vi "Set Up Data Repo.vi"(8 "error in (no error)":errorcluster, 11 "Application in":refnum<class "Application.lvclass">) -> (0 "error out":errorcluster, 3 "Application out":refnum<class "Application.lvclass">)   [LabVIEW 2017, in "Application.lvlib" / "Application.lvclass"]
doc: "Set up the required data header information in the repo."
uses:
  Application.lvclass
  <vilib>/TSS/ACRObat Test Framework/Core Launcher/Core Manager Methods -- Enum.ctl
  <vilib>/TSS/ACRObat Test Framework/Core Launcher/Core Launcher.lvlib
  <vilib>/TSS/ACRObat Test Framework/Classes/Data/Data Repo/Class/Data Repo.lvclass
  Test Recipe/Class/Test Recipe.lvclass
  Station Config/Class/Station Config.lvclass
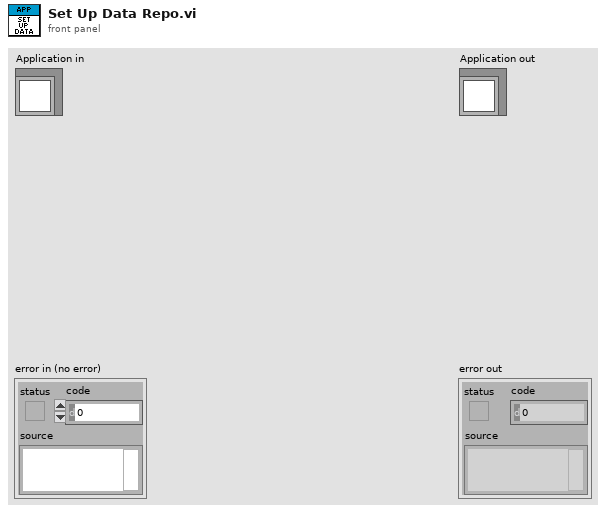
[diagram p1: front panel]
types:
  T1 = typedef "Core Launcher.lvlib/Core Manager Methods -- Enum.ctl" = enum16{"Spawn Objects", "Get Objects", "Destroy Objects"}
  T2 = cluster{"Serial":string, "DateCode":string, "MachID":string, "OperatorID":string, "PartNumber":string, "RecipeFileRev":string, "SoftwareRev":string, "LogField1":string, "LogField2":string, "LogField3":string, "OpMode":string, "PartFailCode":string, "MachineFailCode":string, "Position":string}
  T3 = typedef "Application.lvlib/App Properties.lvclass/Class Properties -- Cluster.ctl" = cluster{"UUT Info":T4[], "Test Information":refnum<vi>, "Gold Board":refnum<class "Golden Board.lvclass">, "Test Recipe":refnum<class "Test Recipe.lvclass">, "Instruments":refnum<class "Instrument.lvclass">[], "Mode":T5, "Test Results":T6[], "Station Config":refnum<class "Station Config.lvclass">, "Variable Engine":refnum<class "Variable Engine.lvclass">}
  T4 = typedef "Application.lvlib/App Properties.lvclass/UUT Reference -- Cluster.ctl" = cluster{"Serial Number Reference":refnum<vi>, "Status Message Reference":refnum<vi>}
  T5 = typedef "Application.lvlib/Application.lvclass/Op Mode -- Enum.ctl" = u16
  T6 = typedef "Application.lvlib/App Properties.lvclass/Test Result -- Cluster.ctl" = cluster{"Position":i32, "Pass":bool, "Fail Codes":string}
  T7 = typedef "Station Config.lvlib/Station Config.lvclass/Station Settings -- Cluster.ctl" = cluster{"Description":string, "ID":string}
  T8 = typedef "Application.lvlib/Application.lvclass/Test Info -- Cluster.ctl" = cluster{"Time / Date":string, "Operator ID":string, "Material":string, "Log Field":string, "Test Time":string, "Software Revision":string}
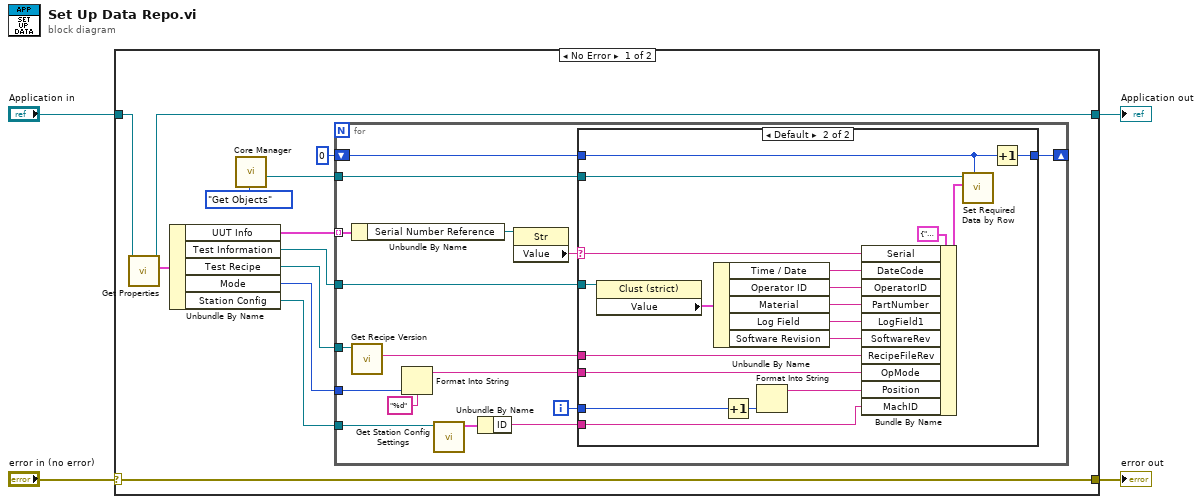
[diagram p0: block diagram]
diagram:
  n1 = case shown="No Error" "error in (no error)" {
    selector: "error in (no error)" -> [w16 w54]
    tunnel: [w16 w54] -> w3
    tunnel: [w14 w53] -> w1
    tunnel: "Application in" -> [w15 w53]
    frame No Error {
      n2 = call "Get Properties.vi"("Acrobat Template in"=w15) -> ("Class Properties"=w13:T3, "Acrobat Template out"=w14:refnum<class "Application.lvclass">)  [unwired: 8 in, 1 out]
      n3 = Unbundle By Name(w13) -> ("UUT Info"=w11:T4[], "Test Information"=w10:refnum<vi>, "Test Recipe"=w7:refnum<class "Test Recipe.lvclass">, "Mode"=w6:T5, "Station Config"=w5:refnum<class "Station Config.lvclass">)
      n4 = call <vilib>:"Core Manager.vi"("Method"=Core_Manager_Methods_--_Enum."Get Objects") -> ("Data Repo"=w12:refnum<class "Data Repo.lvclass">)  [unwired: 6 in, 4 out]
      n5 = for {
        tunnel: w12 -> [w32]
        tunnel: w11 -> [w29] mode=indexing
        tunnel: w10 -> [w30]
        shift-right: [w25] -> _
        shift-left: 0 -> [w26]
        tunnel: w7 -> [w24]
        tunnel: w6 -> [w22]
        tunnel: w5 -> [w19]
        i -> [w27]
        n6 = Unbundle By Name(w29) -> ("Serial Number Reference"=w28:refnum<vi>)
        n7 = call "Get Recipe Version.vi"("Test Recipe in"=w24) -> ("Test Recipe Version"=w23:string)  [unwired: 8 in, 2 out]
        n8 = Format Into String(format string="%d", w22) -> (resulting string=w20:string)  [unwired: 2 in, 1 out]
        n9 = call "Get Station Config Settings.vi"("Station Config in"=w19) -> ("Station Settings"=w18:T7)  [unwired: 9 in, 1 out]
        n10 = Unbundle By Name(w18) -> ("ID"=w17:string)
        n11 = property class="Str"(reference=w28) -> ("Value"=w31:string)  [unwired: 1 in, 2 out]
        n12 = case shown="Default" w31 {
          selector: w31 -> [_ w50]
          tunnel: w32 -> [_ w52]
          tunnel: w30 -> [_ w49]
          tunnel: w27 -> [_ w42]
          tunnel: w26 -> [w33 w39]
          tunnel: [w33 w38] -> w25
          tunnel: w23 -> [_ w36]
          tunnel: w20 -> [_ w37]
          tunnel: w17 -> [_ w34]
          frame "" {
          }
          frame Default {
            n13 = property class="Clust (strict)"(reference=w49) -> ("Value"=w47:T8)  [unwired: 1 in, 2 out]
            n14 = Unbundle By Name(w47) -> ("Time / Date"=w46:string, "Operator ID"=w45:string, "Material"=w44:string, "Log Field"=w43:string, "Software Revision"=w35:string)
            n15 = Increment(x=w42) -> (x+1=w40:i32)
            n16 = Format Into String(w40) -> (resulting string=w41:string)  [unwired: 3 in, 1 out]
            n17 = Bundle By Name(cluster=T2 {"Serial"="", "DateCode"="", "MachID"="", "OperatorID"="", "PartNumber"="", "RecipeFileRev"="", "SoftwareRev"="", "LogField1"="", "LogField2"="", "LogField3"="", "OpMode"="", "PartFailCode"="", "MachineFailCode"="", "Position"=""} ("Required Data"), "Serial"=w50, "DateCode"=w46, "OperatorID"=w45, "PartNumber"=w44, "LogField1"=w43, "SoftwareRev"=w35, "RecipeFileRev"=w36, "OpMode"=w37, "Position"=w41, "MachID"=w34) -> (w48:T2)
            n18 = call <vilib>:"Set Required Data by Row.vi"("Row"=w39, "Required Data"=w48, "Acrobat Template in"=w52) -> ()  [unwired: 7 in, 2 out]
            n19 = Increment(x=w39) -> (x+1=w38:i32)
          }
        }
      }
    }
    frame Error {
    }
  }
  "error out" <- w3
  "Application out" <- w1
